vi "Configure Measurement (Channel Power).vi"(0 "VISA resource name":refnum<visa-resource-name>, 1 "Auto Range (T: Enable)":bool=TRUE, 2 "Top Amplitude (-10 dBm)":dbl=-10.0, 5 "Integration Bandwidth (2E+6 Hz)":dbl=2000000.0, 7 "Channel Power Span (3E+6 Hz)":dbl=3000000.0, 9 "Center Frequency (3.5E+9 Hz)":dbl=3500000000.0, 11 "error in (no error)":errorcluster, 12 "Bottom Amplitude (-70 dBm)":dbl=-70.0) -> (4 "VISA resource name out":refnum<visa-resource-name>, 15 "error out":errorcluster)   [LabVIEW 2022 SP3, in "Agilent N934X Series.lvlib"]
doc: "Sets the Channel Power measurement parameters."
uses:
  <instrlib>/Agilent N934X Series/Agilent N934X Series.lvlib
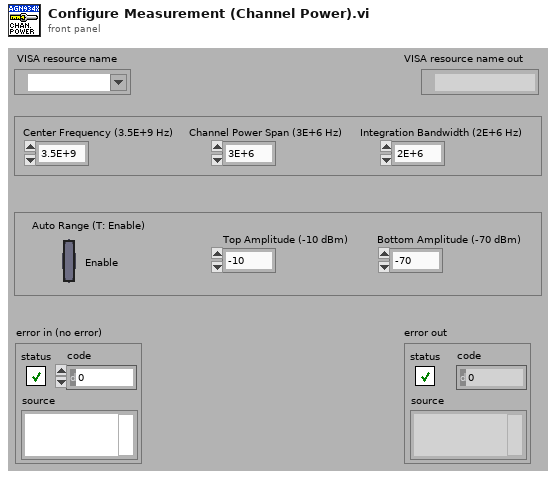
[diagram p1: front panel]
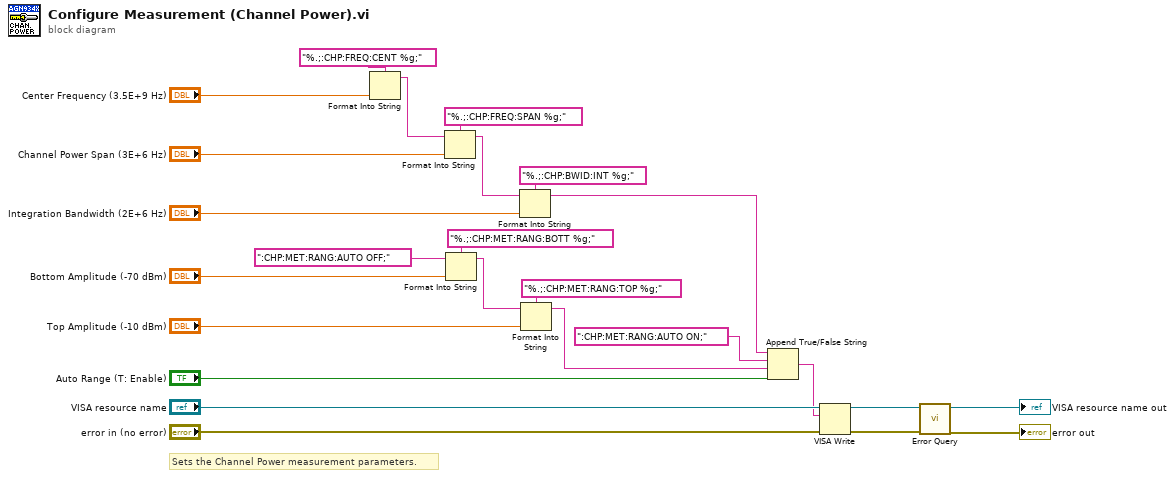
[diagram p0: block diagram]
diagram:
  # "Sets the Channel Power measurement parameters."
  n1 = Format Into String(format string="%.;:CHP:FREQ:CENT %g;", "Center Frequency (3.5E+9 Hz)") -> (resulting string=w23:string)  [unwired: 2 in, 1 out]
  n2 = Format Into String(format string="%.;:CHP:FREQ:SPAN %g;", initial string=w23, "Channel Power Span (3E+6 Hz)") -> (resulting string=w20:string)  [unwired: 1 in, 1 out]
  n3 = Format Into String(format string="%.;:CHP:MET:RANG:BOTT %g;", initial string=":CHP:MET:RANG:AUTO OFF;", "Bottom Amplitude (-70 dBm)") -> (resulting string=w15:string)  [unwired: 1 in, 1 out]
  n4 = Format Into String(format string="%.;:CHP:BWID:INT %g;", initial string=w20, "Integration Bandwidth (2E+6 Hz)") -> (resulting string=w3:string)  [unwired: 1 in, 1 out]
  n5 = Format Into String(format string="%.;:CHP:MET:RANG:TOP %g;", initial string=w15, "Top Amplitude (-10 dBm)") -> (resulting string=w4:string)  [unwired: 1 in, 1 out]
  n6 = Append True/False String(1:"Auto Range (T: Enable)", 2:w4, 3:":CHP:MET:RANG:AUTO ON;", 4:w3) -> (0:w2:string)
  n7 = VISA Write(VISA resource name="VISA resource name", write buffer=w2, error in (no error)="error in (no error)") -> (VISA resource name out=w10:refnum<visa-resource-name>, error out=w9:errorcluster)  [unwired: 1 out]
  n8 = call <instrlib>:"Error Query.vi"("error in (no error)"=w9, "VISA resource name"=w10) -> ("error out"=→"error out":errorcluster, "VISA resource name out"=→"VISA resource name out":refnum<visa-resource-name>)  [unwired: 6 in, 2 out]
